vi "Limit Check and Report.vi"(9 "Expected Value":dbl, 10 "Tolerance (%)":i8, 11 "Last Value":dbl) -> (2 "Report Text":string, 3 "Boolean":bool)   [LabVIEW 2016, in "TLMB.lvlib"]
uses:
  Projects/TLMB.lvlib
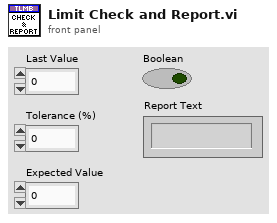
[diagram p1: front panel]
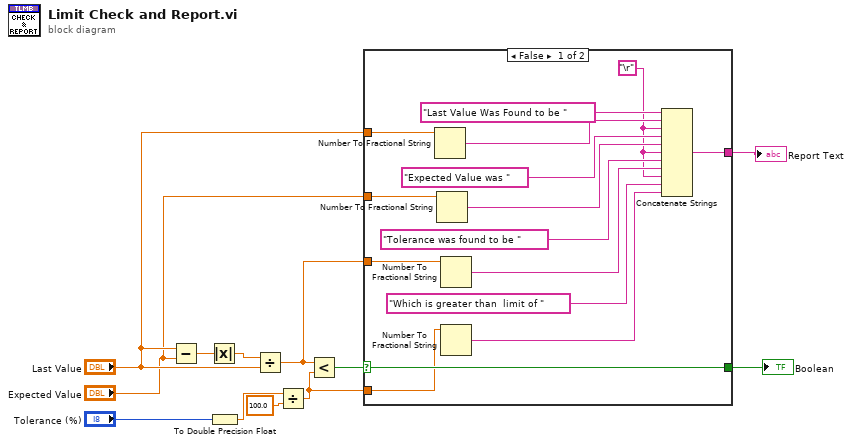
[diagram p0: block diagram]
diagram:
  n1 = Subtract(x="Last Value", y="Expected Value") -> (x-y=w8:dbl)
  n2 = Absolute Value(x=w8) -> (abs(x)=w9:dbl)
  n3 = To Double Precision Float(number="Tolerance (%)") -> (double precision float=w11:dbl)
  n4 = Divide(x=w9, y="Last Value") -> (x/y=w3:dbl)
  n5 = Divide(x=w11, y=100.0) -> (x/y=w2:dbl)
  n6 = Less?(x=w3, y=w2) -> (x < y?=w7:bool)
  n7 = case shown="False" w7 {
    selector: w7 -> [w27 w28]
    tunnel: [w27 w28] -> w6
    tunnel: "Last Value" -> [w25 _]
    tunnel: "Expected Value" -> [w24 _]
    tunnel: w3 -> [w23 _]
    tunnel: w2 -> [w22 _]
    tunnel: [w13 _] -> w1
    frame False {
      w16 = "\r"
      n8 = Number To Fractional String(number=w25) -> (F-format string=w21:string)  [unwired: 3 in]
      n9 = Number To Fractional String(number=w24) -> (F-format string=w19:string)  [unwired: 3 in]
      n10 = Number To Fractional String(number=w23) -> (F-format string=w17:string)  [unwired: 3 in]
      n11 = Number To Fractional String(number=w22) -> (F-format string=w14:string)  [unwired: 3 in]
      n12 = Concatenate Strings("Last Value Was Found to be ", w21, w16, "Expected Value was " ("string"), w19, w16, "Tolerance was found to be " ("string"), w17, w16, "Which is greater than  limit of " ("string"), w14) -> (w13:string)
    }
    frame True {
    }
  }
  "Boolean" <- w6
  "Report Text" <- w1
